vi "PUT Number of Samples.vi"(0 "Number of Samples":dbl) -> ()   [LabVIEW 2013]
uses:
  Action.ctl
  Experimental Parameters FGV Selector.ctl
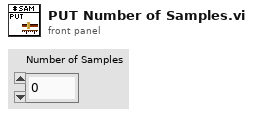
[diagram p1: front panel]
types:
  T1 = typedef "Experimental Parameters FGV Selector.ctl" = enum16{"Number of Samples", "Actuation Direction", "Ramp Rate", "Z Scan Size"}
  T2 = typedef "Action.ctl" = enum16{"GET", "PUT", "DELETE"}
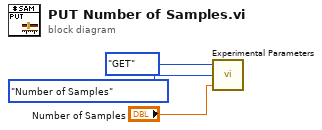
[diagram p0: block diagram]
diagram:
  n1 = call "Experimental Parameters.vi"("Input"="Number of Samples", "Experimental Parameters FGV Selector"=Experimental_Parameters_FGV_Selector."Number of Samples", "Action"=Action."GET") -> ()  [unwired: 1 out]
